vi "BMI.vi"() -> ()   [LabVIEW 2014]
panel:
  in  "stop":bool
  out "BMI":string
  in  "Weight (Kg)":dbl
  out "Result":string
  in  "Height (m)":dbl
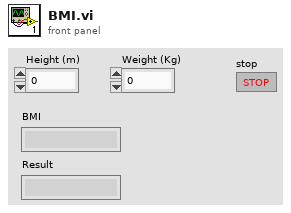
[diagram p1: front panel]
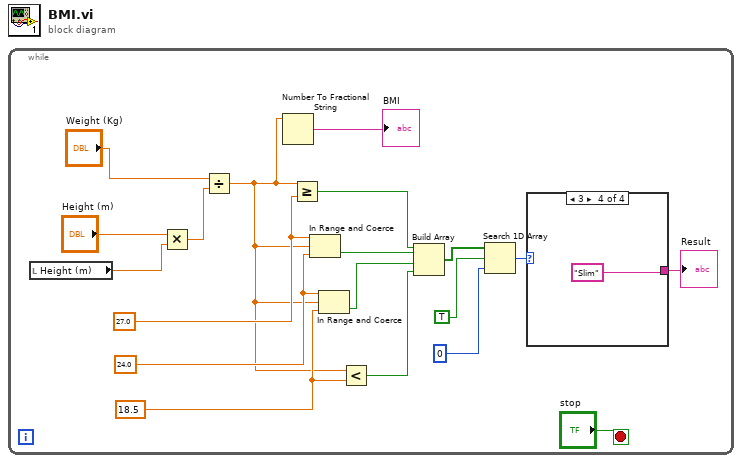
[diagram p0: block diagram]
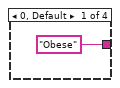
[diagram p2: hidden frame]
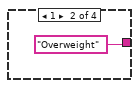
[diagram p3: hidden frame]
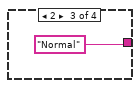
[diagram p4: hidden frame]
diagram:
  n1 = while {
    stop <- "stop" stop-if-true
    w13 = 18.5
    w14 = 24.0
    w15 = 27.0
    n2 = local read "Height (m)"() -> (w19:dbl)
    n3 = Multiply(x="Height (m)", y=w19) -> (x*y=w17:dbl)
    n4 = Divide(x="Weight (Kg)", y=w17) -> (x/y=w12:dbl)
    n5 = Number To Fractional String(number=w12) -> (F-format string=→"BMI":string)  [unwired: 3 in]
    n6 = Greater Or Equal?(x=w12, y=w15) -> (x >= y?=w9:bool)
    n7 = In Range and Coerce(upper limit=w15, x=w12, lower limit=w14) -> (In Range?=w8:bool)  [unwired: 1 out]
    n8 = In Range and Coerce(upper limit=w14, x=w12, lower limit=w13) -> (In Range?=w7:bool)  [unwired: 1 out]
    n9 = Less?(x=w12, y=w13) -> (x < y?=w6:bool)
    n10 = Build Array(w9, w8, w7, w6) -> (w5:bool[])
    n11 = Search 1D Array(1D array=w5, element=TRUE, start index (0)=0) -> (index of element=w2:i32)
    n12 = case shown="3" w2 {
      tunnel: ["Obese" "Overweight" "Normal" "Slim"] -> w1
      frame 0, Default {
      }
      frame 1 {
      }
      frame 2 {
      }
      frame 3 {
      }
    }
    "Result" <- w1
  }
